vi "Contains Mouse.vi"(0 "FSM.Edge":refnum<class "FSM.Edge.lvclass">, 7 "Coords":T1, 9 "threshold":dbl) -> (8 "contains mouse":bool)   [LabVIEW 2020, in "FSM.Edge.lvclass"]
uses:
  FSM.Edge.lvclass
  <vilib>/Utility/miscctls.llb/LVPoint32TypeDef.ctl
  FSM.Edge.lvclass/FSM.Edge.ctl
  FSM.Label/FSM.Label.lvclass
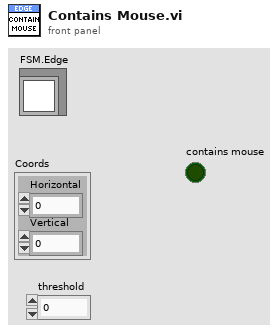
[diagram p1: front panel]
types:
  T1 = typedef "LVPoint32TypeDef.ctl" = cluster{"Horizontal":i32, "Vertical":i32}
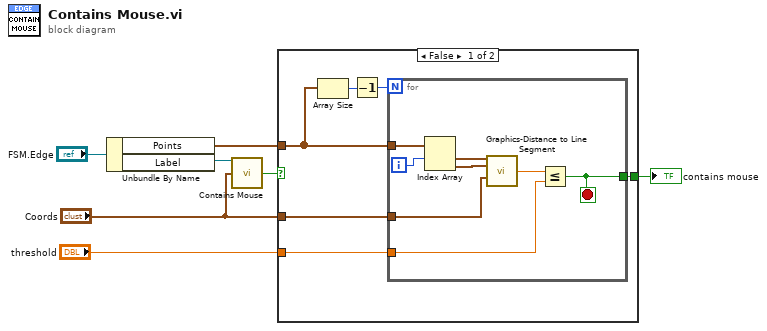
[diagram p0: block diagram]
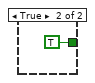
[diagram p2: hidden frame]
diagram:
  n1 = Unbundle By Name("FSM.Edge") -> ("Points"=w6:cluster{"x":i16, "y":i16}[], "Label"=w3:refnum<class "FSM.Label.lvclass">)
  n2 = call "Contains Mouse.vi"("FSM.Label"=w3, "Coords"="Coords") -> ("contains mouse"=w1:bool)  [unwired: 12 in, 1 out]
  n3 = case shown="False" w1 {
    tunnel: w6 -> [w11 _]
    tunnel: "threshold" -> [w10 _]
    tunnel: [w9 TRUE] -> w4
    tunnel: "Coords" -> [w8 _]
    frame False {
      n4 = Array Size(array=w11) -> (size(s)=w13:i32)
      n5 = Decrement(x=w13) -> (x-1=w12:i32)
      n6 = for {
        N: w12 -> [_]
        tunnel: w11 -> [w21]
        tunnel: w8 -> [w17]
        tunnel: w10 -> [w15]
        tunnel: [w14] -> w9
        i -> [w20]
        stop <- w14 stop-if-true
        n7 = Index Array(array=w21, index #1=w20) -> (element #1=w19:cluster{"x":i16, "y":i16}, element #2=w18:cluster{"x":i16, "y":i16})  [unwired: 1 in]
        n8 = call "Graphics-Distance to Line Segment.vi"("segmentStart"=w19, "segmentEnd"=w18, "point"=w17) -> ("distance"=w16:dbl)  [unwired: 12 in]
        n9 = Less Or Equal?(x=w16, y=w15) -> (x <= y?=w14:bool)
      }
    }
    frame True {
    }
  }
  "contains mouse" <- w4
